vi "PTScanner.destructor.vi"(0 "i ref in":refnum<vi>, 5 "error in (no error)":errorcluster) -> (19 "error out":errorcluster)   [LabVIEW 2014, in "PTScanner.lvlib"]
uses:
  PTScanner.lvlib
  CSCore/BaseProcess/BaseProcess.lvlib
  CSCore/BaseGUI/BaseGUI.lvlib
  CSCore/BaseSM/BaseSM.lvlib
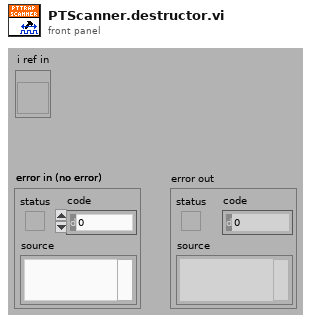
[diagram p1: front panel]
types:
  T1 = typedef "PTScanner.lvlib/PTScanner.i attribute.ctl" = cluster{"Object cmds":T2[], "Steps":cluster{"Finished":bool, "cmd setup":T3[]}[], "curStep":i32, "DIM IDs":cluster{"AllFinished":i32, "Finished":i32, "curStep":i32, "nofSteps":i32, "NomValues":i32[], "1D-Min":i32, "1D-Max":i32, "Dimensions":i32, "MaxDimensions":i32, "ScanedDeviceNames":i32[]}, "All Finished":bool, "DIMs in use":string[], "Running":bool, "Scan Delay":u32, "loop":bool, "Paused":bool, "Formed":bool}
  T2 = typedef "PTScanner.lvlib/PTScanner.obj parameters.ctl" = cluster{"object":string, "DIM address":string, "method":string, "data descriptor":string, "method parameters":cluster{"Name":string, "Descr":string, "Value":string, "Value?":bool}[], "Call Mode":enum16{"Simple DIM", "Synchronous"}, "actValue":dbl, "Centroid":dbl, "Minus Delta":dbl, "Plus Delta":dbl, "increment":dbl, "DIM Status":cluster{"no link":bool, "quality":i32, "Time Stamp":timestamp}, "range":dbl, "DIMChannelIndex":i32}
  T3 = typedef "PTScanner.lvlib/PTScanner.step obj parameters.ctl" = cluster{"obj index":i32, "nomValue":dbl, "fulfilled":bool}
  T4 = enum16{"SetAttribute", "GetAttribute", "CreateAttribute", "DestroyAttribute", "DestroyAllAtributes"}
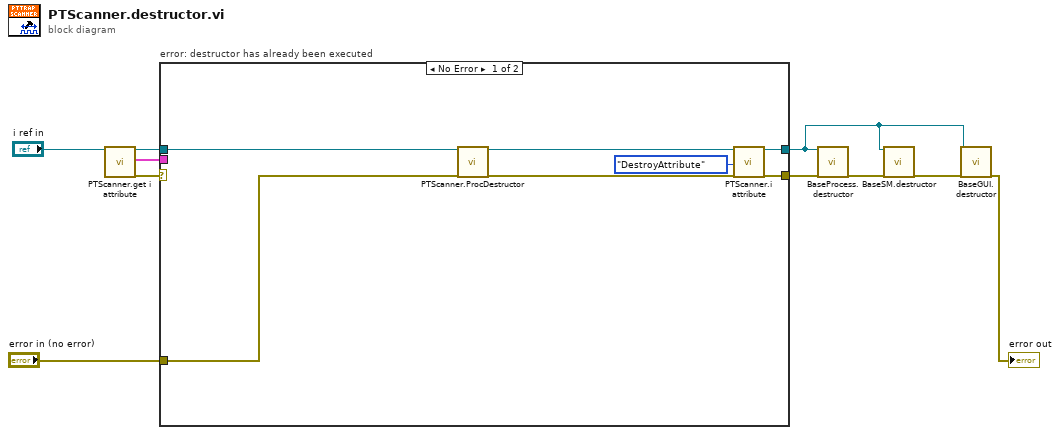
[diagram p0: block diagram]
diagram:
  n1 = call "PTScanner.get i attribute.vi"("i ref in"="i ref in") -> ("i ref out"=w8:refnum<vi>, "i attribute"=w7:T1, "error out"=w9:errorcluster)  [unwired: 16 in]
  n2 = case "error: destructor has already been executed" shown="No Error" w9 {
    selector: w9 -> [_ w18]
    tunnel: w8 -> [w14 w19]
    tunnel: w7 -> [_ _]
    tunnel: [w16 w19] -> w2
    tunnel: [w15 w18] -> w6
    tunnel: "error in (no error)" -> [w11 _]
    frame No Error {
      n3 = call "PTScanner.ProcDestructor.vi"("i ref in"=w14, "error in (no error)"=w11) -> ("i ref out"=w13:refnum<vi>, "error out"=w12:errorcluster)  [unwired: 16 in]
      n4 = call "PTScanner.i attribute.vi"("VI Refnum"=w13, "Action"=T4."DestroyAttribute", "error in (no error)"=w12) -> ("VI Refnum out"=w16:refnum<vi>, "error out"=w15:errorcluster)  [unwired: 14 in, 1 out]
    }
    frame Error {
    }
  }
  n5 = call "BaseProcess.destructor.vi"("i ref in"=w2, "error in (no error)"=w6) -> ("error out"=w4:errorcluster)  [unwired: 17 in]
  n6 = call "BaseSM.destructor.vi"("i ref in"=w2, "error in (no error)"=w4) -> ("error out"=w3:errorcluster)  [unwired: 17 in]
  n7 = call "BaseGUI.destructor.vi"("i ref in"=w2, "error in (no error)"=w3) -> ("error out"=→"error out":errorcluster)  [unwired: 17 in]
